vi "New Time Segmented Log.vi"(8 "error in (no error)":errorcluster, 9 "Max Instances (-1: Unlimited)":i32=-1, 10 "Time Limit [sec]":dbl, 11 "Log File Specification":refnum<class "Log File Specification.lvclass">) -> (0 "error out":errorcluster, 3 "Time Segmented Log out":refnum<class "Time Segmented Log.lvclass">)   [LabVIEW 2015, in "Time Segmented Log.lvclass"]
doc: "Creates a new time-segmented log file, which specifies that a particular log file instance is closed after it has been logged to for a specified amount of time in seconds."
uses:
  Time Segmented Log.lvclass
  Log File Specifications/Log File Specification/Log File Specification.lvclass
  Segmented Log/Segmented Log.lvclass/Segmented Log.ctl
  Time Segmented Log.lvclass/Time Segmented Log.ctl
  Segmented Log/Segmented Log Type.ctl
  Segmented Log/Segmented Log.lvclass
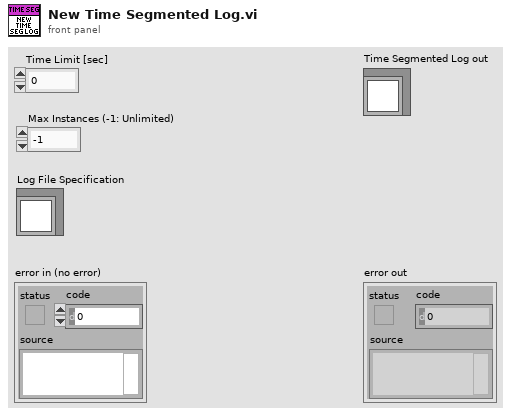
[diagram p1: front panel]
types:
  T1 = typedef "Segmented Log.lvclass/Segmented Log Type.ctl" = enum16{"No Limit", "Footprint", "Time"}
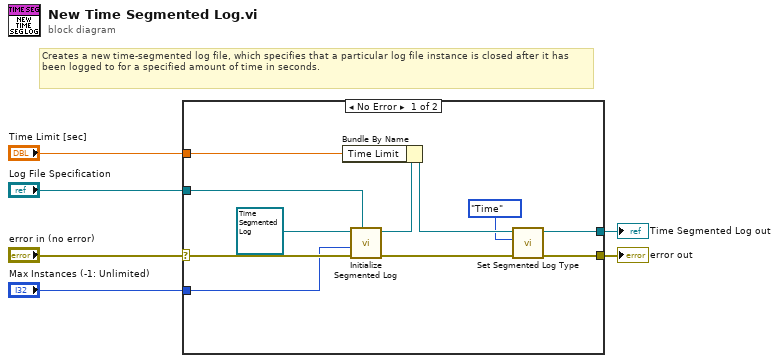
[diagram p0: block diagram]
diagram:
  # "Creates a new time-segmented log file, which specifies that a particular log file instance is closed after it has been logged to for a specified amount of time in seconds."
  n1 = case shown="No Error" "error in (no error)" {
    selector: "error in (no error)" -> [w16 w18]
    tunnel: [w11 w18] -> w5
    tunnel: [w9 _] -> w4
    tunnel: "Log File Specification" -> [w14 _]
    tunnel: "Time Limit [sec]" -> [w13 _]
    tunnel: "Max Instances (-1: Unlimited)" -> [w12 _]
    frame No Error {
      n2 = call "Initialize Segmented Log.vi"("Log File Specification"=w14, "error in (no error)"=w16, "Max Instances (1)"=w12, "Segmented Log in"=refnum<class "Time Segmented Log.lvclass"> refnum ("Time Segmented Log in")) -> ("error out"=w8:errorcluster, "Segmented Log out"=w15:refnum<class "Time Segmented Log.lvclass">)  [unwired: 6 in]
      n3 = Bundle By Name(cluster=w15, "Time Limit"=w13) -> (w10:refnum<class "Time Segmented Log.lvclass">)
      n4 = call "Set Segmented Log Type.vi"("error in (no error)"=w8, "Segmented Log Type"=Segmented_Log_Type."Time", "Segmented Log in"=w10) -> ("error out"=w11:errorcluster, "Segmented Log out"=w9:refnum<class "Time Segmented Log.lvclass">)  [unwired: 7 in]
    }
    frame Error {
    }
  }
  "error out" <- w5
  "Time Segmented Log out" <- w4
